vi "Get Marker Mode.vi"(8 "error in (no error)":errorcluster, 11 "VISA resource name":refnum<visa-resource-name>) -> (0 "error out":errorcluster, 2 "Marker Mode":i32, 3 "VISA resource name out":refnum<visa-resource-name>)   [LabVIEW 2013, in "Fluke 5XXX Series Multicalibrators.lvlib"]
doc: "This VI returns the Marker scope's mode waveform setting.\n\nNote:\n\nThis VI is available only for instrument models 5500A and 5520A with oscilloscope option SC600 (SC1100)."
uses:
  Fluke 5XXX Series Multicalibrators.lvlib
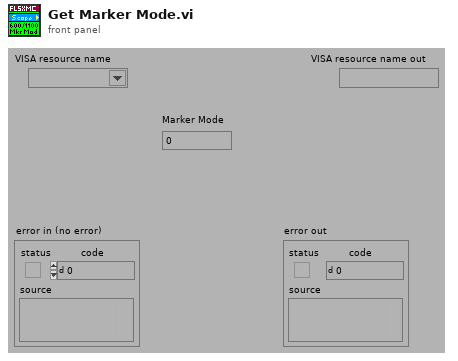
[diagram p1: front panel]
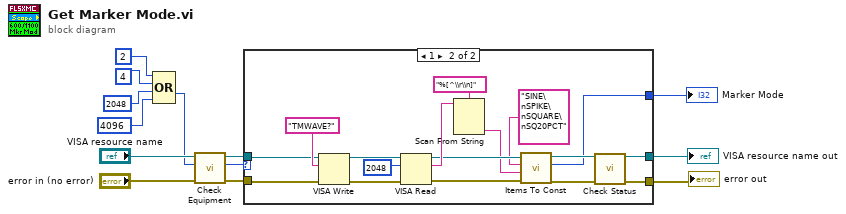
[diagram p0: block diagram]
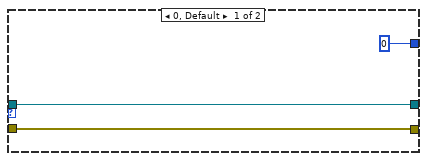
[diagram p2: hidden frame]
diagram:
  n1 = Compound Arithmetic op=OR(2 ("Numeric"), 4 ("Numeric"), 2048 ("Numeric"), 4096 ("Numeric")) -> (w1:i32)
  n2 = call "Check Equipment.vi"("error in (no error)"="error in (no error)", "Bit Mask"=w1, "VISA resource name"="VISA resource name") -> ("error out"=w13:errorcluster, "Present?"=w12:u32, "VISA resource name out"=w11:refnum<visa-resource-name>)  [unwired: 6 in]
  n3 = case shown="1" w12 {
    tunnel: [w16 w27] -> w8
    tunnel: [w15 w26] -> w7
    tunnel: w13 -> [w16 w29]
    tunnel: w11 -> [w15 w28]
    tunnel: [0 w18] -> w6
    frame 0, Default {
    }
    frame 1 {
      n4 = VISA Write(VISA resource name=w28, write buffer="TMWAVE?", error in (no error)=w29) -> (VISA resource name out=w32:refnum<visa-resource-name>, error out=w31:errorcluster)  [unwired: 1 out]
      n5 = VISA Read(VISA resource name=w32, byte count=u32 2048 ("byte count (0)"), error in (no error)=w31) -> (VISA resource name out=w21:refnum<visa-resource-name>, read buffer=w24:string, error out=w22:errorcluster)  [unwired: 1 out]
      n6 = Scan From String(format string="%[^\\r\\n]", input string=w24) -> (output 1=w19:string)  [unwired: 3 in, 3 out]
      n7 = call "Items To Const.vi"("error in (no error)"=w22, "String Item"=w19, "Multi-Line String"="SINE\nSPIKE\nSQUARE\nSQ20PCT", "VISA resource name"=w21) -> ("error out"=w23:errorcluster, "Index"=w18:i32, "VISA resource name out"=w20:refnum<visa-resource-name>)  [unwired: 5 in]
      n8 = call "Check Status.vi"("VISA resource name"=w20, "error in (no error)"=w23) -> ("VISA resource name out"=w26:refnum<visa-resource-name>, "error out"=w27:errorcluster)  [unwired: 12 in]
    }
  }
  "Marker Mode" <- w6
  "VISA resource name out" <- w7
  "error out" <- w8
